vi "next direction.vi"(1 "current direc":i32, 2 "col":i8, 3 "row":i64) -> (0 "next direc":i32)   [LabVIEW 2020]
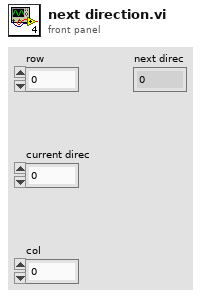
[diagram p1: front panel]
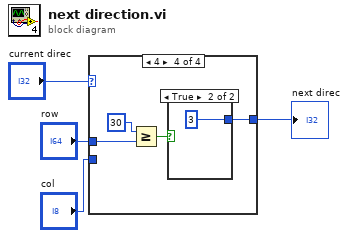
[diagram p0: block diagram]
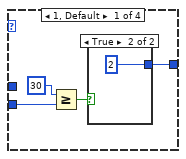
[diagram p2: hidden frame]
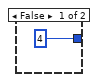
[diagram p3: hidden frame]
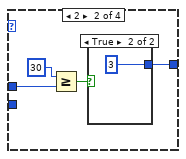
[diagram p4: hidden frame]
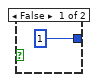
[diagram p5: hidden frame]
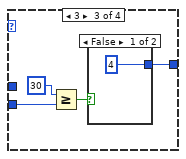
[diagram p6: hidden frame]
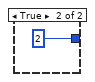
[diagram p7: hidden frame]
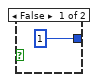
[diagram p8: hidden frame]
diagram:
  n1 = case shown="4" "current direc" {
    tunnel: "col" -> [w7 _ w19 _]
    tunnel: [w5 w12 w17 w24] -> w1
    tunnel: "row" -> [_ w11 _ w23]
    frame 1, Default {
      n2 = Greater Or Equal?(x=i8 30, y=w7) -> (x >= y?=w6:bool)
      n3 = case shown="True" w6 {
        tunnel: [4 2] -> w5
        frame False {
        }
        frame True {
        }
      }
    }
    frame 2 {
      n4 = Greater Or Equal?(x=i8 30, y=w11) -> (x >= y?=w13:bool)
      n5 = case shown="True" w13 {
        tunnel: [1 3] -> w12
        frame False {
        }
        frame True {
        }
      }
    }
    frame 3 {
      n6 = Greater Or Equal?(x=i8 30, y=w19) -> (x >= y?=w18:bool)
      n7 = case shown="False" w18 {
        tunnel: [4 2] -> w17
        frame False {
        }
        frame True {
        }
      }
    }
    frame 4 {
      n8 = Greater Or Equal?(x=i8 30, y=w23) -> (x >= y?=w25:bool)
      n9 = case shown="True" w25 {
        tunnel: [1 3] -> w24
        frame False {
        }
        frame True {
        }
      }
    }
  }
  "next direc" <- w1
